vi "Initialize.vi"(8 "error in (no error)":errorcluster, 11 "BeginJob in":refnum<class "BeginJob.lvclass">) -> (0 "error out":errorcluster, 3 "BeginJob out":refnum<class "BeginJob.lvclass">)   [LabVIEW 2013, in "HardwareCharacterization.lvlib" / "BeginJob.lvclass"]
uses:
  BeginJob.lvclass
  Elements.ctl
  Element-XML.lvclass/Element-XML.ctl
  Write Element.vi
  Element-XML.lvclass
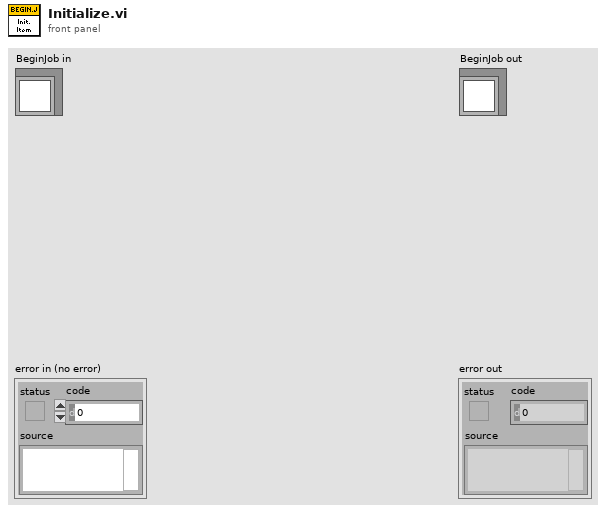
[diagram p1: front panel]
types:
  T1 = typedef "HardwareCharacterization.lvlib/Element-XML.lvclass/Elements.ctl" = enum16{"BeginJob", "WriteDigital", "WriteAnalog", "Set", "ApplicationEvent", "JumpAbs", "MarkAbs", "JumpRel", "MarkRel", "LongDelay", "EndJob"}
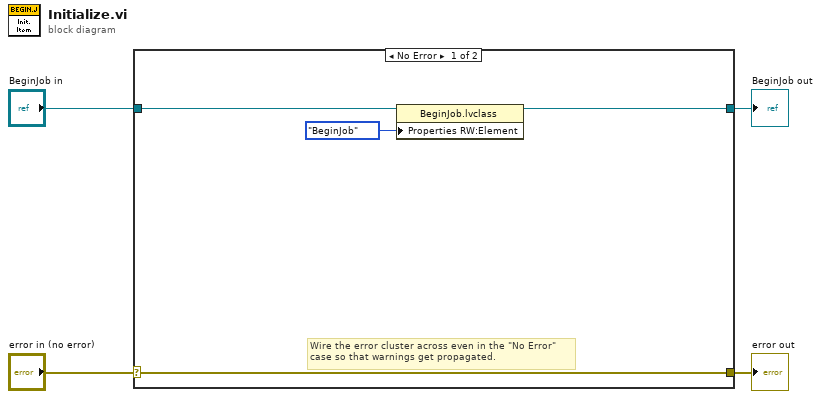
[diagram p0: block diagram]
diagram:
  n1 = case shown="No Error" "error in (no error)" {
    selector: "error in (no error)" -> [w7 w10]
    tunnel: [w7 w10] -> w3
    tunnel: [w6 w9] -> w1
    tunnel: "BeginJob in" -> [w8 w9]
    frame No Error {
      # "Wire the error cluster across even in the \"No Error\"\ncase so that warnings get propagated."
      n2 = property class="BeginJob.lvclass"(reference=w8, "Properties RW:Element"=Elements."BeginJob" ("Element")) -> (reference out=w6:refnum<class "BeginJob.lvclass">)  [unwired: 1 in, 1 out]
    }
    frame Error {
    }
  }
  "error out" <- w3
  "BeginJob out" <- w1
